vi "Voltage_to_unsigned_8bit_3 (SubVI).vi"(11 "Voltage_in":dbl) -> ()   [LabVIEW 2016]
panel:
  out "unsigned 16bit integer":u16
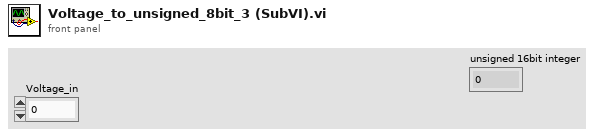
[diagram p1: front panel]
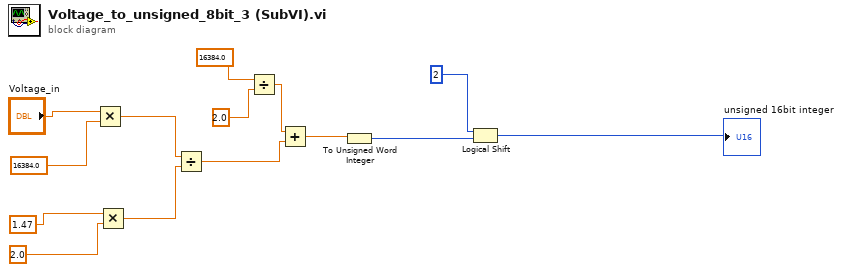
[diagram p0: block diagram]
diagram:
  n1 = Multiply(x="Voltage_in", y=16384.0) -> (x*y=w10:dbl)
  n2 = Multiply(x=1.47, y=2.0) -> (x*y=w9:dbl)
  n3 = Divide(x=w10, y=w9) -> (x/y=w5:dbl)
  n4 = Divide(x=16384.0, y=2.0) -> (x/y=w6:dbl)
  n5 = Add(x=w6, y=w5) -> (x+y=w4:dbl)
  n6 = To Unsigned Word Integer(number=w4) -> (unsigned 16bit integer=w2:u16)
  n7 = Logical Shift(y=2, x=w2) -> (x << y=→"unsigned 16bit integer":u16)
